vi "Z Aux Direct Set Param.vi"(7 "fset":sgl, 8 "error in (no error)":errorcluster caption="错误输入（无错误）", 9 "iaxis":i32, 10 "sParam":string, 11 "handle":u32) -> (0 "error out":errorcluster caption="错误输出", 2 "function return":i32, 3 "handle out":u32)   [LabVIEW 2015, in "zauxdll.lvlib"]
doc: "int32 __stdcall ZAux_Direct_SetParam(ZMC_HANDLE handle,const char *sParam,int iaxis, float fset);"
uses:
  zauxdll.lvlib
  zauxdll.dll
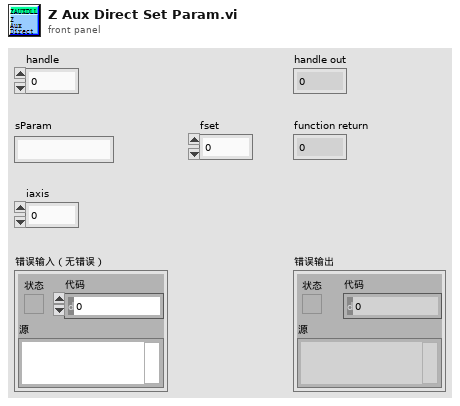
[diagram p1: front panel]
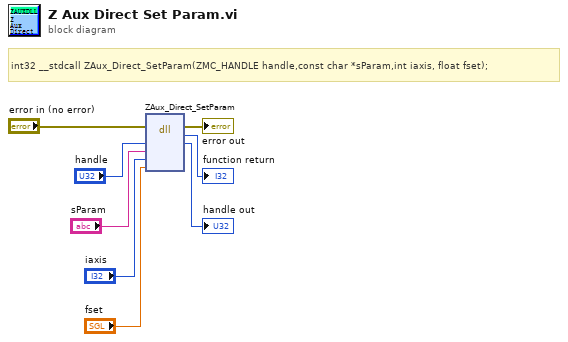
[diagram p0: block diagram]
diagram:
  # "int32 __stdcall ZAux_Direct_SetParam(ZMC_HANDLE handle,const char *sParam,int iaxis, float fset);"
  n1 = dll-call lib="C:/Users/VIC/Desktop/GOGORO_Oringnal - Panasonic/system/LLB/zmotion/zaux/zauxdll.*" fn="ZAux_Direct_SetParam"(error in="error in (no error)", "handle"="handle", "sParam"="sParam", "iaxis"="iaxis", "fset"="fset") -> (error out=→"error out":errorcluster, →"function return":i32, "handle"=→"handle out":u32)  [unwired: 5 in, 1 out]
